vi "picoquant_shove_into_data_queue.vi"(8 "error in (no error)":errorcluster, 10 "new_data":u32[](array[numeric])=[1, 0, 1, 1, 0, 0, 1, 1, 0, 0, 0, 0, 1, 0, 0, 1, 0, 0, 1, 1, 1, 1, 1, 1, 1, 0, 0, 0, 0, 1, 1, 0, 1, 1, 0, 1, 1, 1, 1, 0, 0, 0, 0, 0, 0, 0, 0, 1, 1, 1, 1, 1, 1, 0, 0, 0, 1, 1, 0, 1, 1, 0, 1, 1, 0, 0, 1, 1, 0, 1, 0, 1, 0, 0, 1, 0, 0, 1, 1, 1, 1, 1, 0, 0, 1, 1, 0, 1, 0, 1, 0, 1, 1, 0, 1, 1, 0, 0, 1, 1, 0, 1, 1, 0, 0, 1, 1, 1, 1, 0, 0, 1, 1, 1, 0, 0, 0, 1, 0, 0, 0, 1, 0, 1, 0, 1, 0, 0], 11 "picoquant_generic in":refnum<class "picoquant_generic.lvclass">) -> (0 "error out":errorcluster, 3 "picoquant_generic out":refnum<class "picoquant_generic.lvclass">)   [LabVIEW 2015, in "picoquant_generic.lvclass"]
uses:
  picoquant_generic.lvclass
  picoquant_generic.lvclass/picoquant_generic.ctl
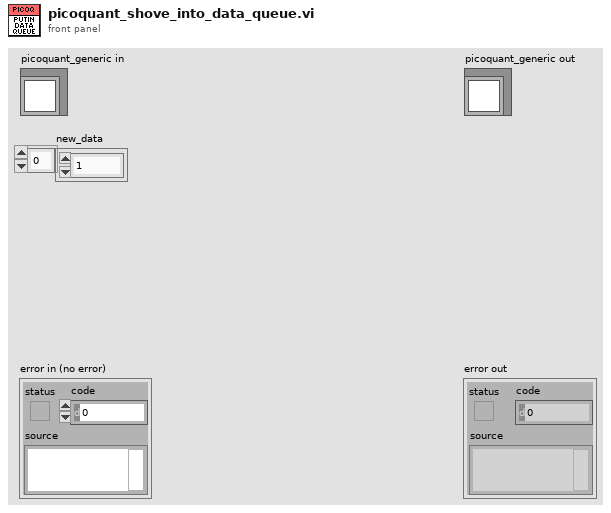
[diagram p1: front panel]
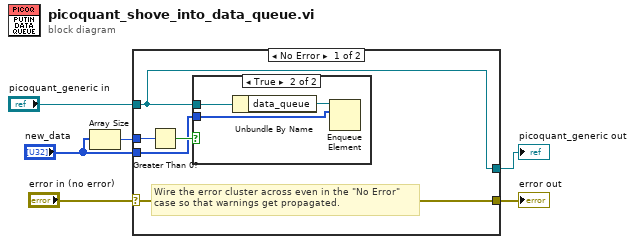
[diagram p0: block diagram]
diagram:
  n1 = Array Size(array="new_data") -> (size(s)=w2:i32)
  n2 = case shown="No Error" "error in (no error)" {
    selector: "error in (no error)" -> [w11 w16]
    tunnel: [w11 w16] -> w5
    tunnel: [w8 w15] -> w3
    tunnel: "picoquant_generic in" -> [w8 w15]
    tunnel: w2 -> [w10 _]
    tunnel: "new_data" -> [w7 _]
    frame No Error {
      # "Wire the error cluster across even in the \"No Error\"\ncase so that warnings get propagated."
      n3 = Greater Than 0?(x=w10) -> (x > 0?=w9:bool)
      n4 = case shown="True" w9 {
        tunnel: w8 -> [_ w14]
        tunnel: w7 -> [_ w12]
        frame False {
        }
        frame True {
          n5 = Unbundle By Name(w14) -> ("data_queue"=w13:refnum<queue>)
          n6 = Enqueue Element(queue=w13, element=w12) -> ()  [unwired: 2 in, 3 out]
        }
      }
    }
    frame Error {
    }
  }
  "error out" <- w5
  "picoquant_generic out" <- w3
